vi "WOS.vi"(0 "System no.":i32=1 min=1 max=4 step=1, 2 "Generator ID":i32[](array[numeric]) min=1 step=1, 3 "Offset":dbl[](array[numeric]) format="%_6g", 4 "No.of digits":i16=4, 5 "error in":errorcluster) -> (19 "error out":errorcluster)   [LabVIEW 2020]
doc: "Sets wave generator output offset. The current wave generator output is created by adding the output offset value to the current wave value:\nGenerator Output = Output Offset + Current Wave Value.\nThe value is also modified by the generator when the WGO command was executed with iStartMod bit 8 set: At the end of each cycle the output offset value is equate with the current Generator Output. No. of digits is the number of digits after the decimal point in the offset value(s) that will be sent.\n\nC-413: Generator ID can be 1 to 2.\n\nE-517, E-518: Generator ID can be 1 to 3. You can set the offset also using the CFG wave type (see WAV command) or by directly changing the Wave Offset parameter, ID 0x1300010b, with SPA.\n\nE-709: Generator ID can be 1\n\nE-712: Generator ID can be 1 to No. of connected axes\n\nE-725, E-727: Generator ID can be 1 to No. of connected axes\n\nE-753: Generator ID can be 1\n\nE-754: Generator ID can be 1"
panel:
  # "Sets Wave Generator Output Offset."
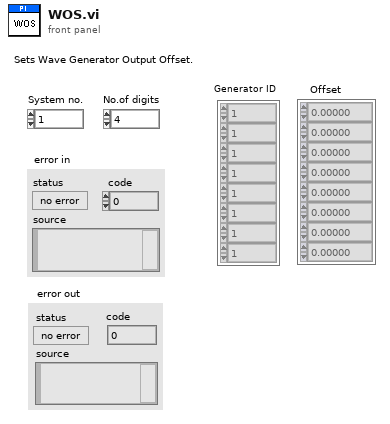
[diagram p1: front panel]
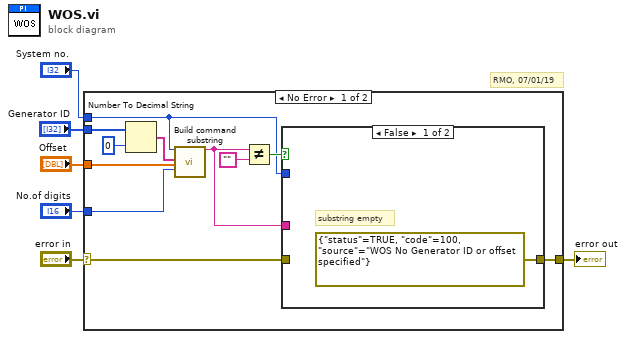
[diagram p0: block diagram]
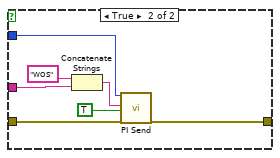
[diagram p2: hidden frame]
diagram:
  # "RMO, 07/01/19"
  n1 = case shown="No Error" "error in" {
    selector: "error in" -> [w7 w26]
    tunnel: [w17 w26] -> w6
    tunnel: "Offset" -> [w14 _]
    tunnel: "System no." -> [w12 _]
    tunnel: "Generator ID" -> [w10 _]
    tunnel: "No.of digits" -> [w8 _]
    frame No Error {
      n2 = Number To Decimal String(number=w10, width (-)=i16 0) -> (decimal integer string=w11:string[])
      n3 = call "Build command substring.vi"("System no."=w12, "Affected axes"=w11, "Parameters"=w14, "No. of digits"=w8) -> ("Command substring"=w15:string)  [unwired: 3 in, 12 out]
      n4 = Not Equal?(x=w15, y="") -> (x != y?=w13:bool)
      n5 = case shown="False" w13 {
        tunnel: w15 -> [_ w24]
        tunnel: [errorcluster {"status"=TRUE, "code"=100, "source"="WOS No Generator ID or offset specified"} ("error out") w19] -> w17
        tunnel: w7 -> [_ w21]
        tunnel: w12 -> [_ w20]
        frame False {
          # "substring empty"
        }
        frame True {
          n6 = Concatenate Strings("WOS", w24) -> (w22:string)
          n7 = call "PI Send.vi"("System no."=w20, "String to send"=w22, "Attach termination char.?"=TRUE ("Attach Linefeed?"), "error in"=w21) -> ("error out"=w19:errorcluster)  [unwired: 2 in, 13 out]
        }
      }
    }
    frame Error {
    }
  }
  "error out" <- w6
